vi "Teleop.vi"(10 "Match Info":T1={"Autonomous Elapsed Seconds"=0.0, "TeleOp Elapsed Seconds"=0.0, "Disabled Elapsed Seconds"=0.0, "Visited Autonomous"=FALSE, "Visited TeleOp"=FALSE, "Visited Disabled"=FALSE, "Autonomous Settings"={"Autonomous Style"=enum."Independent", "VI Refnum"=refnum}}, 11 "Call Context":T2) -> ()   [LabVIEW 2019]
doc: "This VI is called for each TeleOp packet received from the DS where the robot is not disabled. It is often used to read from the joysticks and update I/O or to update setpoints for timed control loops. It should complete and return within 20 milliseconds or it may miss DS packets."
uses:
  <vilib>/Rock Robotics/WPI/DriverStation/WPI_DriverStationDerivedRobotMode.ctl
  <vilib>/Rock Robotics/WPI/DriverStation/WPI_DriverStationMatch Info.ctl
  Typedefs/typedef_enum_TeleOp_State.ctl
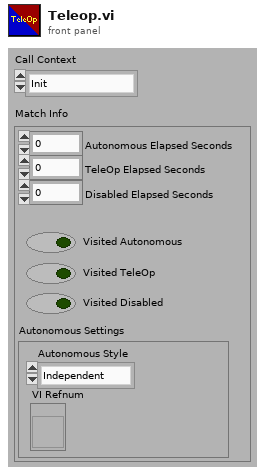
[diagram p1: front panel]
types:
  T1 = typedef "WPI_DriverStationMatch Info.ctl" = cluster{"Autonomous Elapsed Seconds":dbl, "TeleOp Elapsed Seconds":dbl, "Disabled Elapsed Seconds":dbl, "Visited Autonomous":bool, "Visited TeleOp":bool, "Visited Disabled":bool, "Autonomous Settings":cluster{"Autonomous Style":enum16{"Iterative", "Independent"}, "VI Refnum":refnum<vi>}}
  T2 = typedef "WPI_DriverStationDerivedRobotMode.ctl" = enum16{"Init", "Execute", "Stop"}
  T3 = typedef "typedef_enum_TeleOp_State.ctl" = enum16{"Read_Joy", "Calc_Drive", "Write_Drive"}
  T4 = typedef "typedef_cluster_TeleOp_Local_Data.ctl" = cluster{"JoyStick_L":T5, "JoyStick_R":T5, "Drive_Forward":dbl, "Drive_Twist":dbl}
  T5 = typedef "typedef_cluster_Joystick.ctl" = cluster{"X":dbl, "Y":dbl, "Z":dbl, "Throttle":dbl, "Trigger":bool, "Thumb":bool, "Top 3":bool, "Top 4":bool, "Top 5":bool, "Top 6":bool, "Bottom 7":bool, "Bottom 8":bool, "Bottom 9":bool, "Bottom 10":bool, "Bottom 11":bool, "Bottom 12":bool}
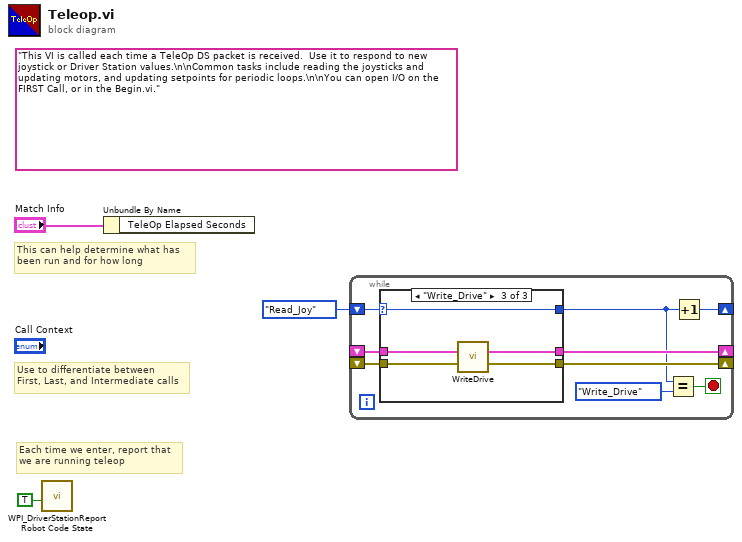
[diagram p0: block diagram]
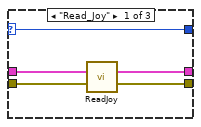
[diagram p2: hidden frame]
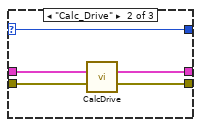
[diagram p3: hidden frame]
diagram:
  (unwired) "This VI is called each time a TeleOp DS packet is received.  Use it to respond to new joystick or Driver Station values.\n\nCommon tasks include reading the joysticks and updating motors, and updating setpoints for periodic loops.\n\nYou can open I/O on the FIRST Call, or in the Begin.vi."
  # "Each time we enter, report that\nwe are running teleop"
  # "Use to differentiate between\nFirst, Last, and Intermediate calls"
  # "This can help determine what has\nbeen run and for how long"
  n1 = call <vilib>:"WPI_DriverStationReport Robot Code State.vi"("TeleOp"=TRUE ("Autonomous")) -> ()  [unwired: 10 in, 1 out]
  n2 = Unbundle By Name("Match Info") -> ()  [unwired: 1 out]
  n3 = while {
    shift-right: [w9] -> _
    shift-left: typedef_enum_TeleOp_State."Read_Joy" ("Enum") -> [w10]
    shift-right: [w5] -> _
    shift-left: _ -> [w8]
    shift-right: [w6] -> _
    shift-left: _ -> [w7]
    stop <- w12 stop-if-true
    n4 = case shown="\"Write_Drive\"" w10 {
      selector: w10 -> [w17 w21 w26]
      tunnel: [w17 w21 w26] -> w4
      tunnel: w8 -> [w16 w20 w25]
      tunnel: w7 -> [w15 w18 w24]
      tunnel: [w14 w18 w22] -> w6
      tunnel: [w13 w19 w23] -> w5
      frame "Read_Joy" {
        n5 = call "ReadJoy.vi"("Teleop Local Data In"=w16, "error in (no error)"=w15) -> ("Teleop Local Data Out"=w13:T4, "error out"=w14:errorcluster)  [unwired: 12 in]
      }
      frame "Calc_Drive" {
        n6 = call "CalcDrive.vi"("Teleop Local Data In"=w20) -> ("Teleop Local Data Out"=w19:T4)  [unwired: 14 in]
      }
      frame "Write_Drive" {
        n7 = call "WriteDrive.vi"("Teleop Local Data In"=w25, "error in"=w24) -> ("Teleop Local Data Out"=w23:T4, "error out"=w22:errorcluster)  [unwired: 12 in]
      }
    }
    n8 = Equal?(x=w4, y=typedef_enum_TeleOp_State."Write_Drive" ("Enum")) -> (x = y?=w12:bool)
    n9 = Increment(x=w4) -> (x+1=w9:T3)
  }
